vi "simple.vi"() -> (3 "Numeric":i32)   [LabVIEW 2012]
uses:
  Global.vi
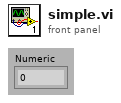
[diagram p1: front panel]
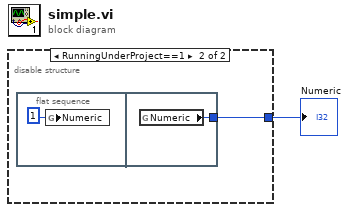
[diagram p0: block diagram]
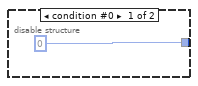
[diagram p2: hidden frame]
diagram:
  n1 = disable-structure shown="RunningUnderProject==1" {
    disable-tunnel: [0 w3] -> w1
    frame condition #0 {
    }
    frame condition #1 (active) {
      n2 = flat-sequence {
        tunnel: [w5] -> w3
        frame #0 {
          n3 = global write "Global.vi" "Numeric"(1 ("Numeric")) -> ()
        }
        frame #1 {
          n4 = global read "Global.vi" "Numeric"() -> (w5:i32)
        }
      }
    }
  }
  "Numeric" <- w1
